vi "Engine-RPC-HPVCtrl.vi"(0 "Control Enable":bool, 1 "Fault Input":bool, 2 "RailP Setpoint":sgl, 3 "Battery [V]":sgl, 11 "Output Management Controls":T2, 13 "Open Loop DC Table":cluster{"XArray":sgl[], "YArray":sgl[]}) -> (4 "Output":T1={"Current_Calc"=0.0, "DutyCyc_TblOut"=0.7671859, "DutyCyc_MaxCalc"=0.0, "DutyCyc_Des"=0.7671859}, 15 "LS Output":T3)   [LabVIEW 2016, in "DSI-RT.lvlib"]
uses:
  DSI-RT.lvlib
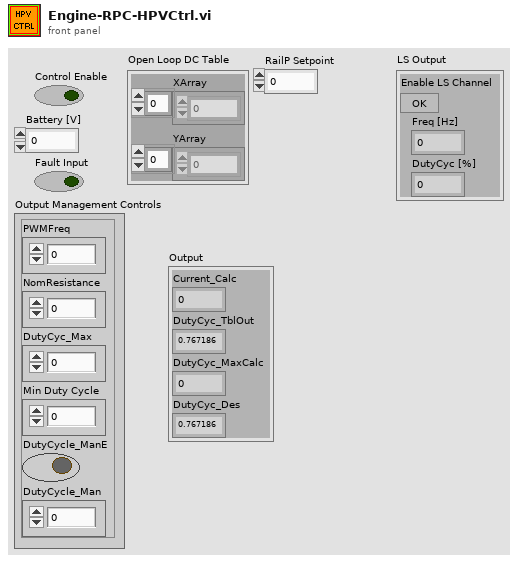
[diagram p1: front panel]
types:
  T1 = cluster{"Current_Calc":sgl, "DutyCyc_TblOut":sgl, "DutyCyc_MaxCalc":sgl, "DutyCyc_Des":sgl}
  T2 = cluster{"PWMFreq":sgl, "NomResistance":sgl, "DutyCyc_Max":sgl, "Min Duty Cycle":sgl, "DutyCycle_ManE":bool, "DutyCycle_Man":sgl}
  T3 = cluster{"Enable LS Channel":bool, "Freq [Hz]":sgl, "DutyCyc [%]":sgl}
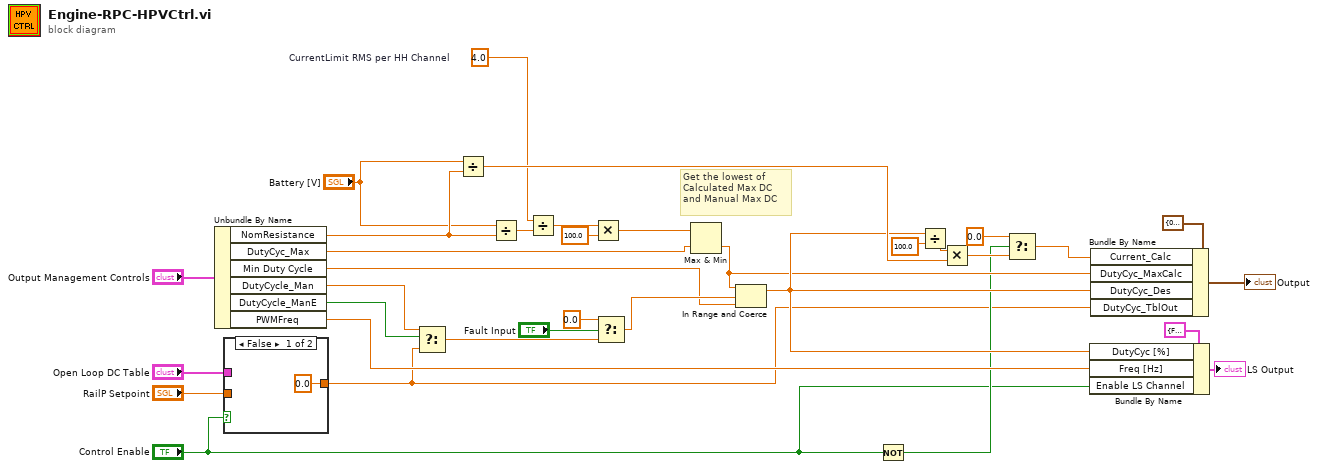
[diagram p0: block diagram]
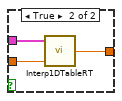
[diagram p2: hidden frame]
diagram:
  w12 = sgl 4.0  # CurrentLimit RMS per HH Channel
  # "Get the lowest of \nCalculated Max DC\nand Manual Max DC"
  n1 = Unbundle By Name("Output Management Controls") -> ("NomResistance"=w16:sgl, "DutyCyc_Max"=w14:sgl, "Min Duty Cycle"=w21:sgl, "DutyCycle_Man"=w20:sgl, "DutyCycle_ManE"=w19:bool, "PWMFreq"=w17:sgl)
  n2 = case shown="False" "Control Enable" {
    tunnel: "Open Loop DC Table" -> [_ w38]
    tunnel: [sgl 0.0 ("Y") w37] -> w7
    tunnel: "RailP Setpoint" -> [_ w36]
    frame False {
    }
    frame True {
      n3 = call <vilib>:"Interp1DTableRT.vi"("X"=w36, "1DTable"=w38) -> ("Y"=w37:sgl)  [unwired: 1 in]
    }
  }
  n4 = Select(t=w20, s=w19, f=w7) -> (s? t:f=w24:sgl)
  n5 = Divide(x="Battery [V]", y=w16) -> (x/y=w31:sgl)
  n6 = Divide(x="Battery [V]", y=w16) -> (x/y=w30:sgl)
  n7 = Divide(x=w12, y=w30) -> (x/y=w29:sgl)
  n8 = Multiply(x=w29, y=sgl 100.0) -> (x*y=w15:sgl)
  n9 = Select(t=sgl 0.0, s="Fault Input", f=w24) -> (s? t:f=w23:sgl)
  n10 = Max & Min(x=w15, y=w14) -> (min(x,y)=w13:sgl)  [unwired: 1 out]
  n11 = In Range and Coerce(upper limit=w13, x=w23, lower limit=w21) -> (coerced(x)=w18:sgl)  [unwired: 1 out]
  n12 = Not(x="Control Enable") -> (.not. x?=w9:bool)
  n13 = Divide(x=w18, y=sgl 100.0) -> (x/y=w32:sgl)
  n14 = Multiply(x=w32, y=w31) -> (x*y=w34:sgl)
  n15 = Select(t=sgl 0.0, s=w9, f=w34) -> (s? t:f=w22:sgl)
  n16 = Bundle By Name(cluster=T3 {"Enable LS Channel"=FALSE, "Freq [Hz]"=0.0, "DutyCyc [%]"=0.0} ("LS Output"), "DutyCyc [%]"=w18, "Freq [Hz]"=w17, "Enable LS Channel"="Control Enable") -> (→"LS Output":T3)
  n17 = Bundle By Name(cluster=T1 {"Current_Calc"=0.0, "DutyCyc_TblOut"=0.7671859, "DutyCyc_MaxCalc"=0.0, "DutyCyc_Des"=0.7671859} ("HPV"), "Current_Calc"=w22, "DutyCyc_MaxCalc"=w13, "DutyCyc_Des"=w18, "DutyCyc_TblOut"=w7) -> (→"Output":T1)
